vi "picoharp_update_xy_graph_with_correlation.vi"(8 "error in (no error)":errorcluster, 11 "hydraharp in":refnum<class "picoharp.lvclass">) -> (0 "error in (no error) 2":errorcluster, 3 "hydraharp in 2":refnum<class "picoharp.lvclass">)   [LabVIEW 2015, in "picoharp.lvclass"]
uses:
  picoharp.lvclass
  picoharp.lvclass/picoharp.ctl
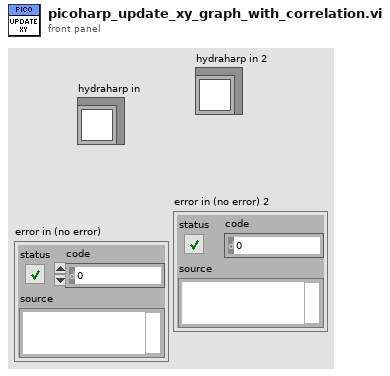
[diagram p1: front panel]
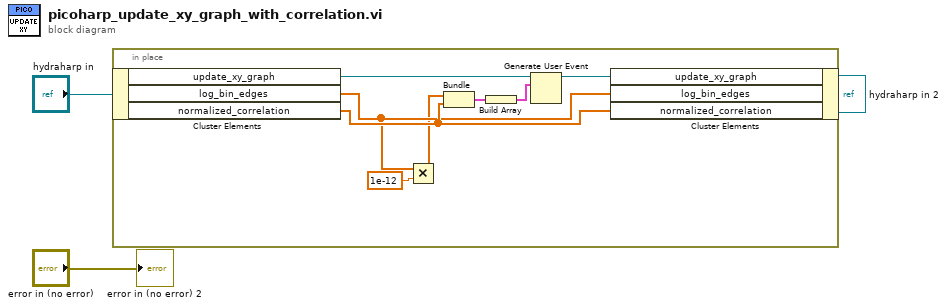
[diagram p0: block diagram]
diagram:
  n1 = in-place {
    n2 = in-place-cluster #1("hydraharp in") -> ("update_xy_graph"=w10:refnum<user-event>, "log_bin_edges"=w5:dbl[], "normalized_correlation"=w7:dbl[])
    n3 = Multiply(x=w5, y=1e-12) -> (x*y=w4:dbl[])
    n4 = Bundle(w4, "normalized_correlation"=w7) -> (w11:cluster{dbl[], "normalized_correlation":dbl[]})  [unwired: 1 in]
    n5 = Build Array(w11) -> (w9:cluster{dbl[], "normalized_correlation":dbl[]}[])
    n6 = Generate User Event(user event=w10, event data cluster=w9) -> (user event out=w8:refnum<user-event>)  [unwired: 2 in, 1 out]
    n7 = in-place-cluster #1("update_xy_graph"=w8, "log_bin_edges"=w5, "normalized_correlation"=w7) -> (→"hydraharp in 2":refnum<class "picoharp.lvclass">)
  }
  "error in (no error) 2" <- "error in (no error)"
